vi "host.vi"() -> ()   [LabVIEW 2020]
uses:
  <vilib>/Analysis/baseanly.llb/Real A x B.vi
  <vilib>/Analysis/Matrix/Numeric/Conversions/Matrix To Array - RM.vi
  <vilib>/FPGAPlugInAG/cRIO-9035/niLvFpga_Open_cRIO-9035.vi
  <vilib>/rvi/interface/common/dynamic/niFpgaDynamicAddResources.vi
  <vilib>/Utility/error.llb/Error Cluster From Error Code.vi
  <vilib>/rvi/errors/niLvFpgaAdjustHostInterfaceError.vi
  <vilib>/FPGAPlugInAG/Dynamic/niLvFpga_Run_Dynamic.vi
  <vilib>/FPGAPlugInAG/Dynamic/niLvFpga_Close_Dynamic.vi
  <vilib>/rvi/interface/nirviOpenFPGA/nirviOpenFPGA.xnode
  FPGA Bitfiles/v1.2_FPGATarget_target_q2D6CmCLiY4.lvbitx
  target.vi
  <vilib>/rvi/interface/nirviMethod/nirviMethod.xnode
  <vilib>/rvi/interface/nirviCloseFPGA/nirviCloseFPGA.xnode
  <vilib>/FPGAPlugInAG/Dynamic/niLvFpga_WriteFifo_Dynamic.vi
  <vilib>/rvi/errors/niLvFpgaMergeErrorWithErrorCode.vi
  <vilib>/Analysis/NI_AALBase.lvlib
  <vilib>/Analysis/Matrix/NI_Matrix.lvlib
  <vilib>/FPGAPlugInAG/Dynamic/niLvFpga_ReadFifo_Dynamic.vi
panel:
  out "elements in B":i32
  out "elements in A":i32
  out "sum of error":dbl
  out "C - FPGA code":sgl[][](array[numeric])
  out "elements in C":i32
  out "C - Real":dbl[][](array[numeric])
  out "B":sgl[][](array[numeric])
  out "A":sgl[][](array[numeric])
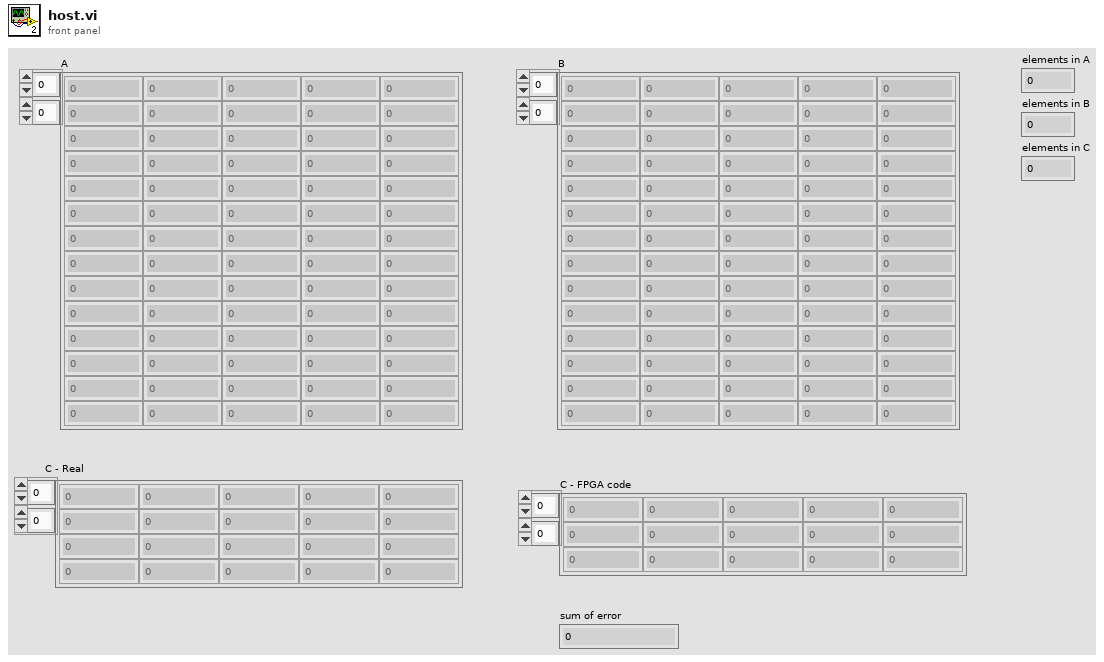
[diagram p1: front panel]
types:
  T1 = typedef "NI_Matrix.lvlib/RealMatrix.ctl" = dbl[][]
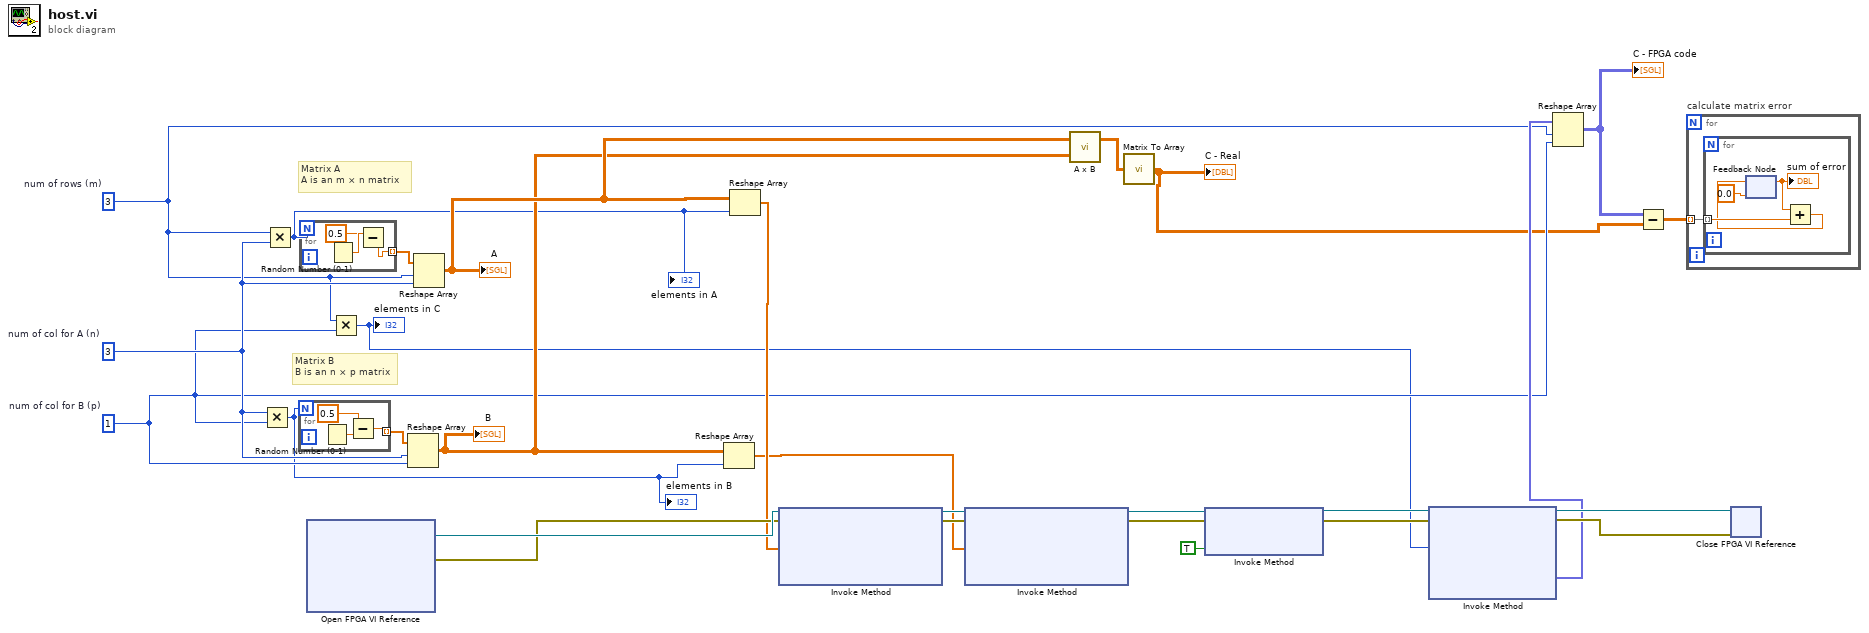
[diagram p0: block diagram]
diagram:
  w4 = 1  # num of col for B (p)
  w11 = 3  # num of col for A (n)
  w5 = 3  # num of rows (m)
  # "Matrix B\nB is an n × p matrix"
  # "Matrix A\nA is an m × n matrix"
  n1 = Multiply(x=w11, y=w4) -> (x*y=w1:i32)
  "elements in B" <- w1
  n2 = Multiply(x=w5, y=w11) -> (x*y=w12:i32)
  "elements in A" <- w12
  n3 = for {
    N: w1 -> [_]
    tunnel: [w30] -> w16 mode=indexing
    n4 = Random Number (0-1)() -> (number: 0 to 1=w31:dbl)
    n5 = Subtract(x=w31, y=sgl 0.5) -> (x-y=w30:sgl)
  }
  n6 = for {
    N: w12 -> [_]
    tunnel: [w33] -> w17 mode=indexing
    n7 = Random Number (0-1)() -> (number: 0 to 1=w34:dbl)
    n8 = Subtract(x=w34, y=sgl 0.5) -> (x-y=w33:sgl)
  }
  n9 = xnode "Open FPGA VI Reference"() -> ("FPGA VI Reference Out"=w27:refnum<k20>, "error out"=w26:errorcluster)  [unwired: 2 in]
  n10 = Multiply(x=w5, y=w4) -> (x*y=w2:i32)
  "elements in C" <- w2
  n11 = Reshape Array(w16, w11, w4) -> (w14:sgl[][])
  "B" <- w14
  n12 = Reshape Array(w17, w5, w11) -> (w15:sgl[][])
  "A" <- w15
  n13 = Reshape Array(w14, w1) -> (w9:sgl[])
  n14 = Reshape Array(w15, w12) -> (w10:sgl[])
  n15 = xnode "Invoke Method"("FPGA VI Reference In"=w27, "error in"=w26, "Data"=w10) -> ("FPGA VI Reference Out"=w21:refnum<k20>, "error out"=w20:errorcluster)  [unwired: 1 in, 1 out]
  n16 = xnode "Invoke Method"("FPGA VI Reference In"=w21, "error in"=w20, "Data"=w9) -> ("FPGA VI Reference Out"=w19:refnum<k20>, "error out"=w18:errorcluster)  [unwired: 1 in, 1 out]
  n17 = call-poly <vilib>:"A x B.vi"("B"=w14, "A"=w15) -> ("A x B"=w13:T1)  [unwired: 1 out]
  n18 = call-poly <vilib>:"Matrix To Array.vi"("Real Matrix"=w13) -> ("Real 2D Array"=w3:dbl[][])
  "C - Real" <- w3
  n19 = xnode "Invoke Method"("FPGA VI Reference In"=w19, "error in"=w18, "Wait Until Done (F)"=TRUE) -> ("FPGA VI Reference Out"=w25:refnum<k20>, "error out"=w24:errorcluster)
  n20 = xnode "Invoke Method"("FPGA VI Reference In"=w25, "error in"=w24, "Number of Elements"=w2) -> ("FPGA VI Reference Out"=w23:refnum<k20>, "error out"=w22:errorcluster, "Data"=w6:fxp<+/-,10,5>[])  [unwired: 1 in, 1 out]
  n21 = Reshape Array(w6, w5, w4) -> (w8:fxp<+/-,10,5>[][])
  "C - FPGA code" <- w8
  n22 = Subtract(x=w8, y=w3) -> (x-y=w7:dbl[][])
  n23 = for "calculate matrix error" {
    tunnel: w7 -> [w35] mode=indexing
    n24 = for {
      tunnel: w35 -> [w39] mode=indexing
      n25 = feedback #1(0.0) -> (w37:dbl)
      "sum of error" <- w37
      n26 = Add(x=w37, y=w39) -> (x+y=w38:dbl)
      n27 = feedback-in #1(w38) -> ()
    }
  }
  n28 = xnode "Close FPGA VI Reference"("FPGA VI Reference In"=w23, "error in"=w22) -> ()  [unwired: 1 out]
